vi "get_safe_path.vi"(8 "error in":errorcluster, 9 "end_label":string, 10 "start_label":string, 11 "filename":string) -> (0 "error out":errorcluster, 2 "coordinates":cluster{"x":dbl, "y":dbl, "z":dbl}[](array[cluster]))   [LabVIEW 2011, in "gVision.lvlib"]
uses:
  gVision.lvlib
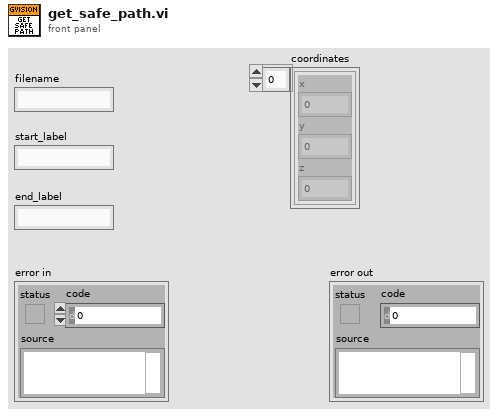
[diagram p1: front panel]
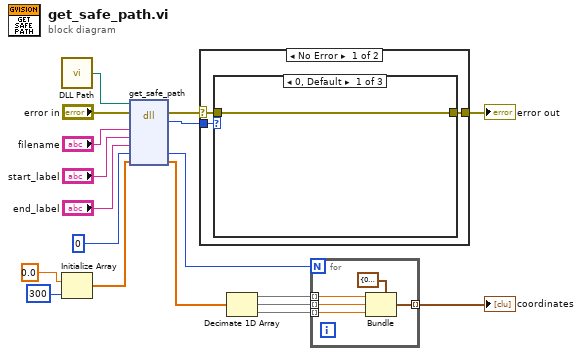
[diagram p0: block diagram]
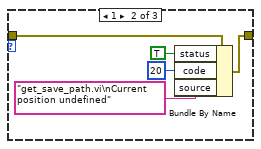
[diagram p2: hidden frame]
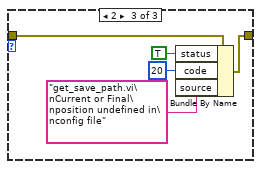
[diagram p3: hidden frame]
diagram:
  n1 = call "DLL Path.vi"() -> ("DLL Path"=w10:path)  [unwired: 5 in]
  n2 = Initialize Array(sgl 0.0 ("element"), 300 ("dimension size")) -> (w16:sgl[])
  n3 = dll-call lib="?" fn="get_safe_path"(path in=w10, error in="error in", "filename"="filename", "start_label"="start_label", "end_label"="end_label", "num_points"=0, "coordinate_list"=w16) -> (error out=w9:errorcluster, "error code"=w8:i32, "num_points"=w6:i32, "coordinate_list"=w5:sgl[])  [unwired: 4 in, 1 out]
  n4 = case shown="No Error" w9 {
    selector: w9 -> [w20 w33]
    tunnel: w8 -> [w21 _]
    tunnel: [w19 w33] -> w7
    frame No Error {
      n5 = case shown="0, Default" w21 {
        tunnel: w20 -> [w22 w27 w29]
        tunnel: [w22 w26 w28] -> w19
        frame 0, Default {
        }
        frame 1 {
          n6 = Bundle By Name(cluster=w27, "status"=TRUE, "code"=20, "source"="get_save_path.vi\nCurrent position undefined") -> (w26:errorcluster)
        }
        frame 2 {
          n7 = Bundle By Name(cluster=w29, "status"=TRUE, "code"=20, "source"="get_save_path.vi\nCurrent or Final\nposition undefined in\nconfig file") -> (w28:errorcluster)
        }
      }
    }
    frame Error {
    }
  }
  "error out" <- w7
  n8 = Decimate 1D Array(w5) -> (w4:sgl[], w3:sgl[], w2:sgl[])
  n9 = for {
    N: w6 -> [_]
    tunnel: w4 -> [w38] mode=indexing
    tunnel: w3 -> [w37] mode=indexing
    tunnel: w2 -> [w36] mode=indexing
    tunnel: [w34] -> w1 mode=indexing
    n10 = Bundle(cluster=cluster{"x":dbl, "y":dbl, "z":dbl} {"x"=0.0, "y"=0.0, "z"=0.0}, "x"=w38, "y"=w37, "z"=w36) -> (w34:cluster{"x":dbl, "y":dbl, "z":dbl})
  }
  "coordinates" <- w1
